vi "thermo_config_dialog.vi"(8 "error in":errorcluster, 11 "thermo in":T1={"type"=enum."COMET Tx5xx (ethernet)", "comment"="", "tag"="", "refresh"=5.0, "IP"="", "port"=502, "VISA"="", "last readout"=timestamp(0 s since 1904-01-01), "TCP ref"=refnum, "VISA sess"="", "idn"="", "press"=0.0, "RH"=0.0, "temp"=0.0, "pres cor"=[], "RH cor"=[], "temp cor"=[], "try left"=0, "failed"=FALSE, "RTD set"=[], "RTD inv"=[], "range"=0.0, "net mode"=enum."MODBUS", "try fail"=enum."Stop trying - return NaN", "timeout [s]"=0.0, "max retries"=0, "sim t [deg]"=0.0, "status"=0} {"status" items=["ok", "retry", "failed"]; "RTD inv" format="%.1f"; "RTD set" format="%.1f"; "temp cor" format="%.1f"; "RH cor" format="%.1f"; "pres cor" format="%.1f"; "refresh" min=0.1 max=1000.0 format="%.2f"}) -> (0 "error out":errorcluster, 3 "thermo out":T1={"type"=enum."COMET Tx5xx (ethernet)", "comment"="", "tag"="", "refresh"=5.0, "IP"="", "port"=502, "VISA"="", "last readout"=timestamp(0 s since 1904-01-01), "TCP ref"=refnum, "VISA sess"="", "idn"="", "press"=0.0, "RH"=0.0, "temp"=0.0, "pres cor"=[], "RH cor"=[], "temp cor"=[], "try left"=0, "failed"=FALSE, "RTD set"=[], "RTD inv"=[], "range"=0.0, "net mode"=enum."MODBUS", "try fail"=enum."Stop trying - return NaN", "timeout [s]"=0.0, "max retries"=0, "sim t [deg]"=0.0, "status"=0} {"status" items=["ok", "retry", "failed"]; "RTD inv" format="%.1f"; "RTD set" format="%.1f"; "temp cor" format="%.1f"; "RH cor" format="%.1f"; "pres cor" format="%.1f"; "refresh" min=0.1 max=1000.0 format="%.2f"})   [LabVIEW 2020]
doc: "Thermometer configuration dialogue."
uses:
  thermo_types.ctl
  Thermometer Config Tab Control.ctl
  Thermometer Fail Action.ctl
  RTD/RTD_preset.ctl
  thermo.ctl
  varilib/varilib.lvlib
panel:
  in  "btn default":bool caption="OK Button"
  in  "tc base":enum32{"Page"}(tab)
  in  "refresh":dbl=30.0 caption="Refresh rate [s]" min=0.0 max=1000.0 format="%#.2f"
  in  "comment":string="dummy thermometer" caption="Instrument comment"
  in  "tag":string="dut" caption="Instrument tag"
  in  "type":T2 caption="Type"
  in  "tc com":enum32{"Page"}(tab)
  in  "timeout":dbl=5.0 caption="Readout timeout [s]" min=0.1 max=30.0
  in  "retry N":i32=10 caption="Maximum readout tries" min=0 max=100
  in  "try fail":T3=enum."Stop trying - return NaN" caption="Retries failed action"
  in  "tc idn":enum32{"Page"}(tab)
  out "ID string":string
  out "temp":string caption="t [deg C]"
  out "RH":string caption="RH [%]"
  out "press":string caption="p [Pa]"
  out "RTD list":T4[](array[typedef]) {"tref" format="%.3f"; "Rref [Ohm]" format="%.3f"; "RTD poly" format="%_6e"}
  out "tc setup":T5
  in  "sim t [deg]":dbl caption="mean t [deg]"
  in  "temp cor":dbl[][](array[numeric]) caption="Temperature corrections [deg C]" format="%.1f"
  in  "IP":string="192.168.2.34" caption="IP address"
  in  "port":u16=502 caption="MODBUS port"
  in  "RH cor":dbl[][](array[numeric]) caption="RH corrections [%]" format="%.1f"
  in  "pres cor":dbl[][](array[numeric]) caption="Pressure corrections [Pa]" format="%.1f"
  in  "btn dmm auto":bool
  in  "tref [deg C]":dbl caption="t ref [deg C]" format="%.3f"
  in  "save btn":bool
  in  "R ref [Ohm]":dbl=100.0 format="%_6f"
  in  "VISA":refnum<visa-resource-name>
  in  "def btn":bool
  in  "rtd sens":u16(ring) caption="Default presets" items=["KT210", "KT210", "Pt100", "Pt1000", "Pt100_PT4"]
  in  "RTD poly":dbl[](array[numeric])=[1.0, 0.005485, 6.65e-06, 0.0, 2.805e-11, 0.0, -2e-17] caption="Polynome [deg C^-n]" format="%_6e"
  in  "load btn":bool
  in  "RTD name":string caption="New preset name"
  in  "range":dbl caption="Range [Ohm]" format="%#_6f"
  out "read ok":bool caption="READ"
  out "read fail":bool
  in  "btn cancel":bool
  in  "btn tst":bool
  in  "btn ok":bool
  # "ref. temp.:"
  # "correction:"
  # "ref. RH.:"
  # "correction:"
  # "ref. pres.:"
  # "correction:"
  # "RTD coefficients:"
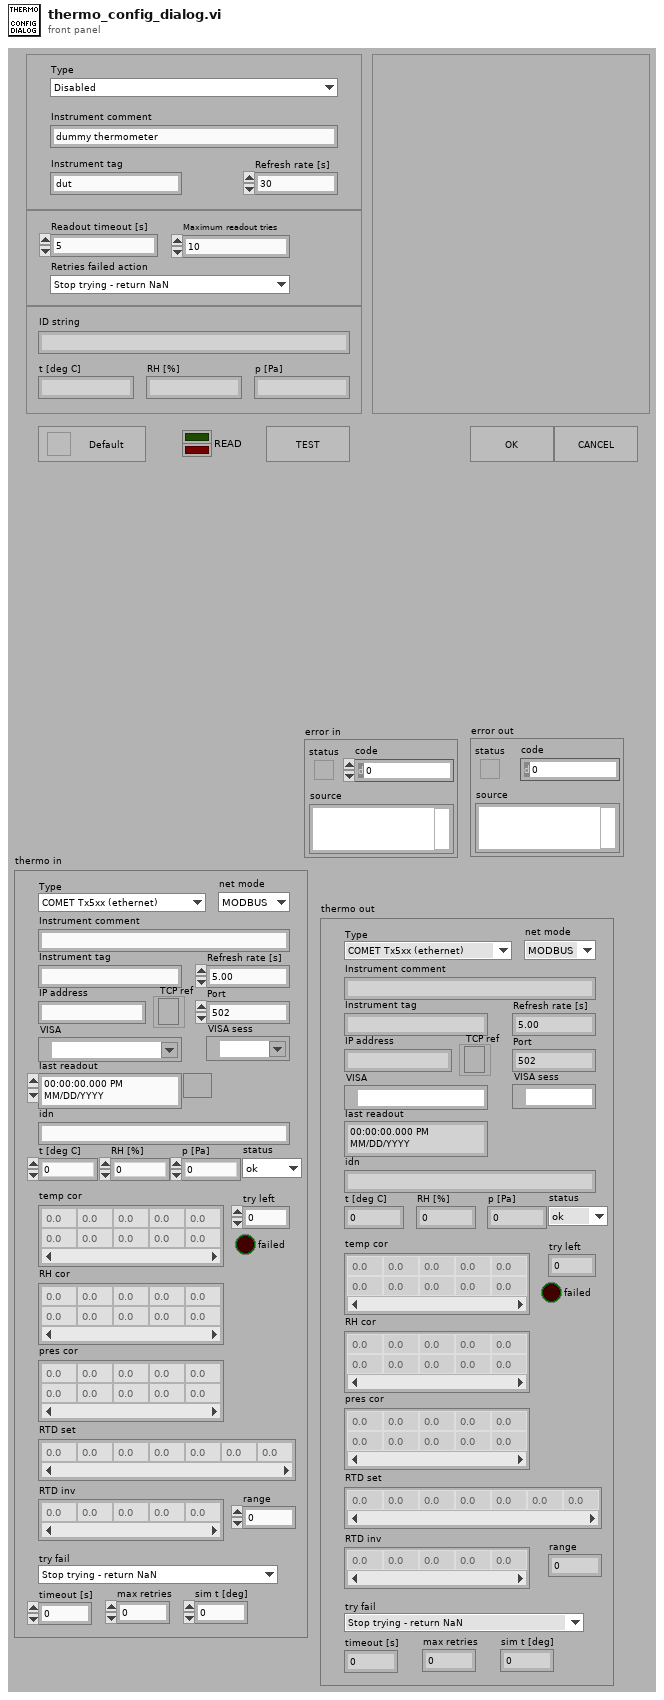
[diagram p1: front panel]
types:
  T1 = typedef "thermo.ctl" = cluster{"type":T2, "comment":string, "tag":string, "refresh":dbl, "IP":string, "port":u16, "VISA":refnum<visa-resource-name>, "last readout":timestamp, "TCP ref":refnum<k5>, "VISA sess":refnum<visa-resource-name>, "idn":string, "press":dbl, "RH":dbl, "temp":dbl, "pres cor":dbl[][], "RH cor":dbl[][], "temp cor":dbl[][], "try left":i32, "failed":bool, "RTD set":dbl[], "RTD inv":dbl[], "range":dbl, "net mode":enum16{"MODBUS", "HTTP"}, "try fail":T3, "timeout [s]":dbl, "max retries":i32, "sim t [deg]":dbl, "status":u16}
  T2 = typedef "thermo_types.ctl" = enum16{"Disabled", "Simulated", "COMET Tx5xx (ethernet)", "Keithley 2002 (GPIB) + RTD", "Agilent 344xx (GPIB) + RTD"}
  T3 = typedef "Thermometer Fail Action.ctl" = enum16{"Stop trying - keep last value", "Stop trying - return NaN", "Generate error - stop sweep"}
  T4 = typedef "RTD_preset.ctl" = cluster{"Rref [Ohm]":dbl, "tref":dbl, "RTD poly":dbl[], "name":string}
  T5 = typedef "Thermometer Config Tab Control.ctl" = enum32{"none", "sim", "COMET", "DMM"}
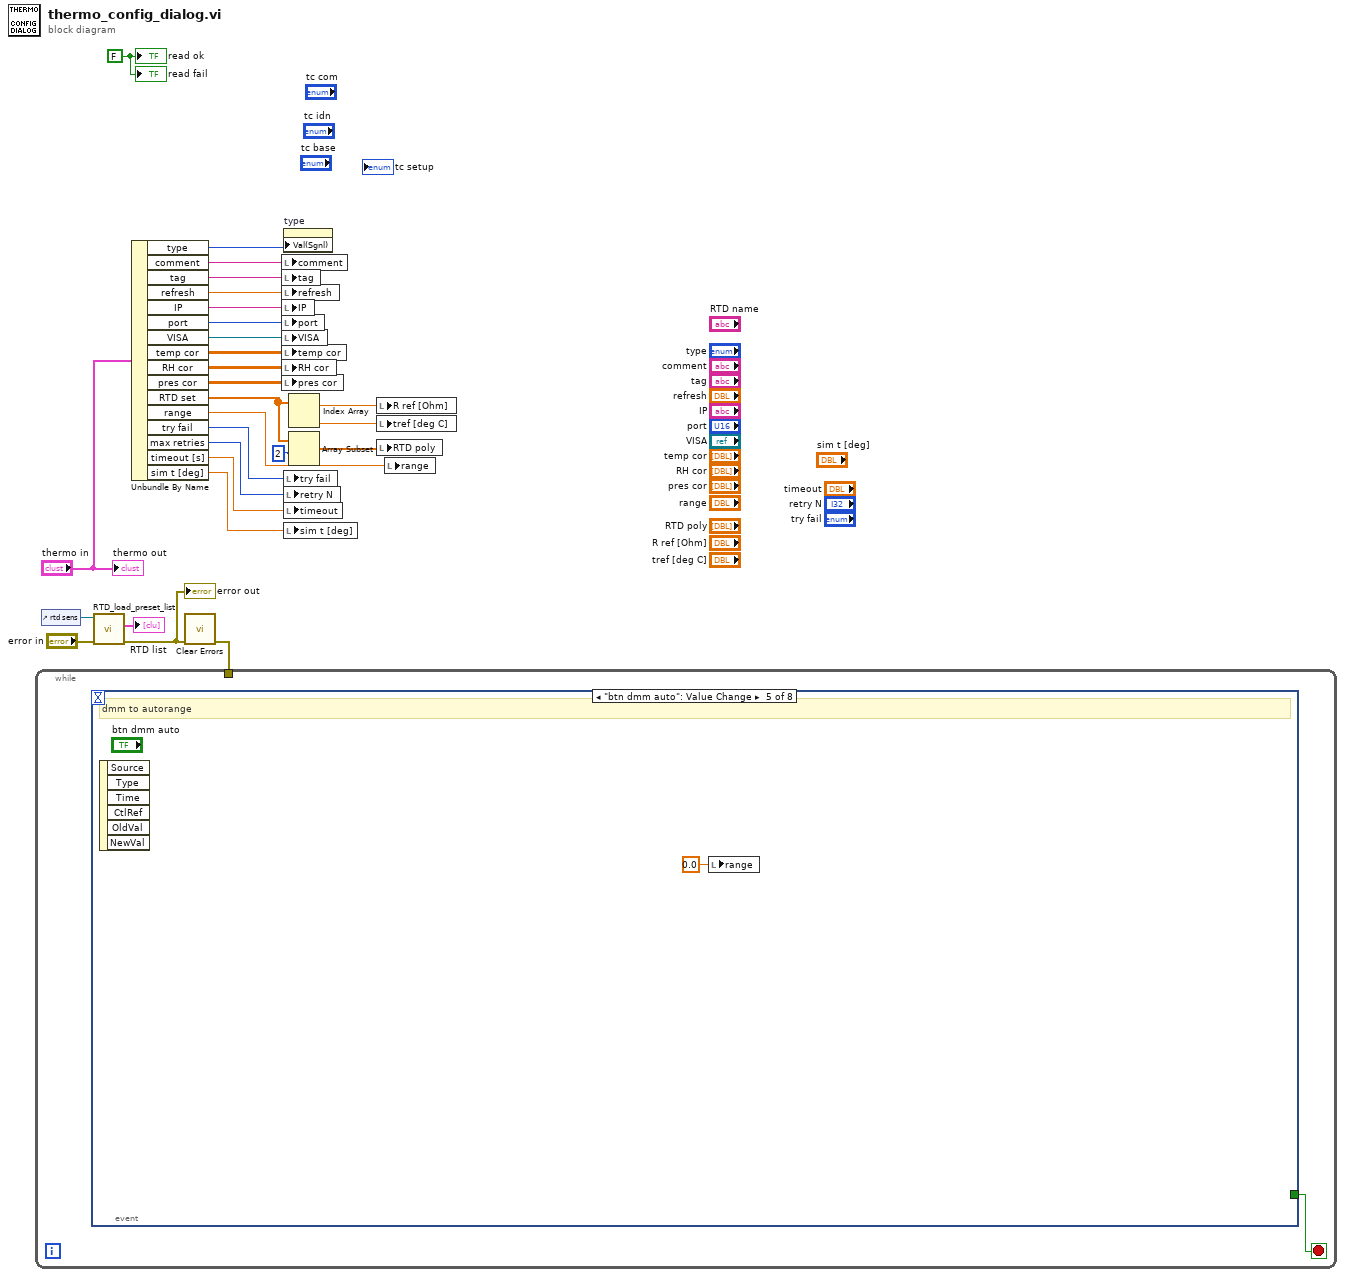
[diagram p0: block diagram]
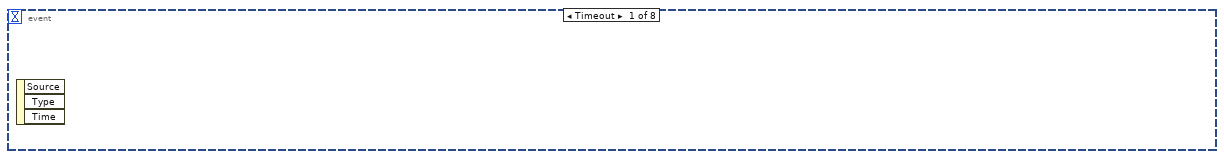
[diagram p2: hidden frame]
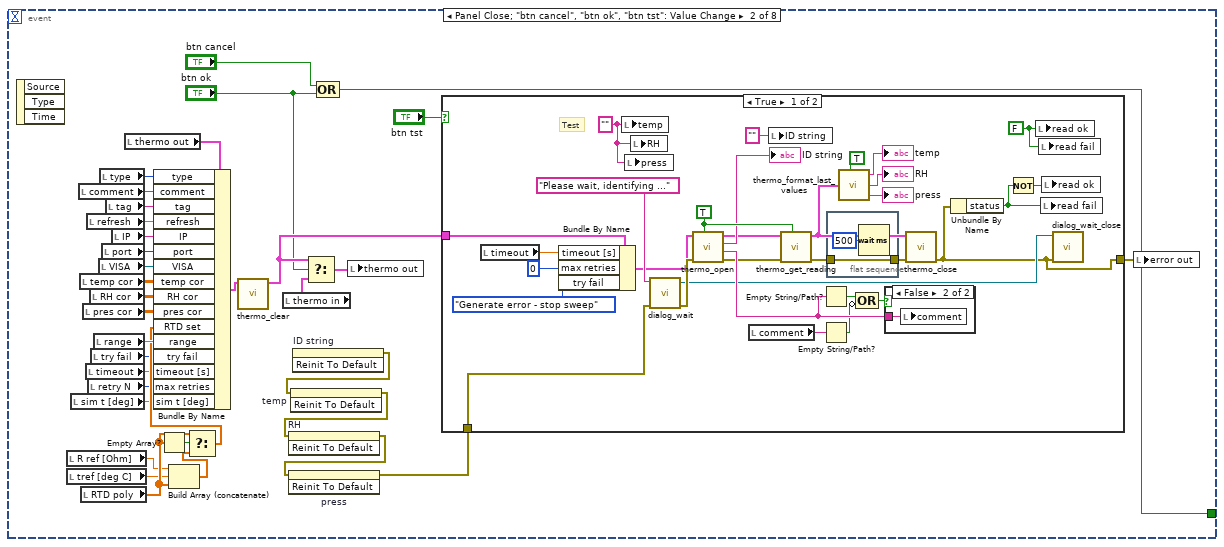
[diagram p3: hidden frame]
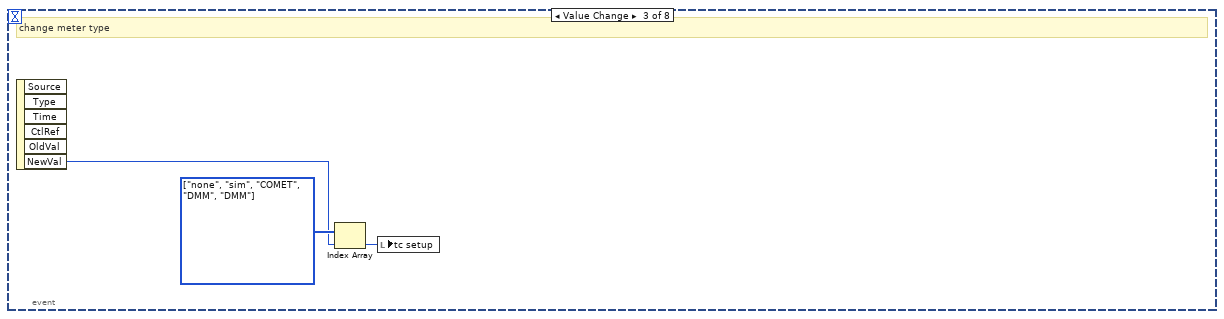
[diagram p6: hidden frame]
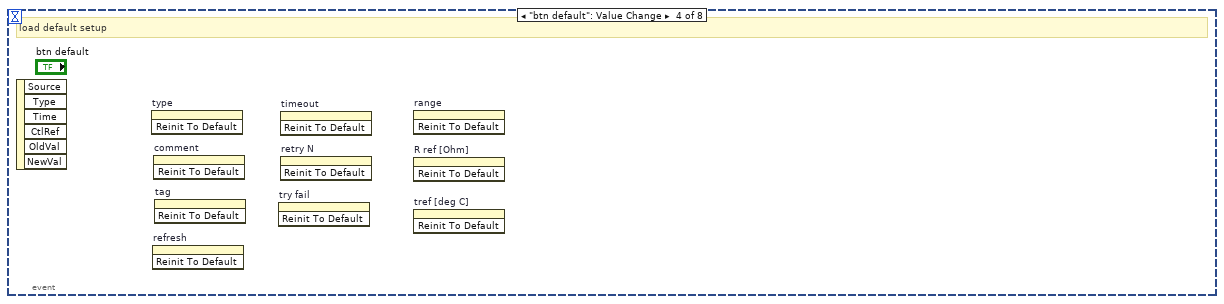
[diagram p7: hidden frame]
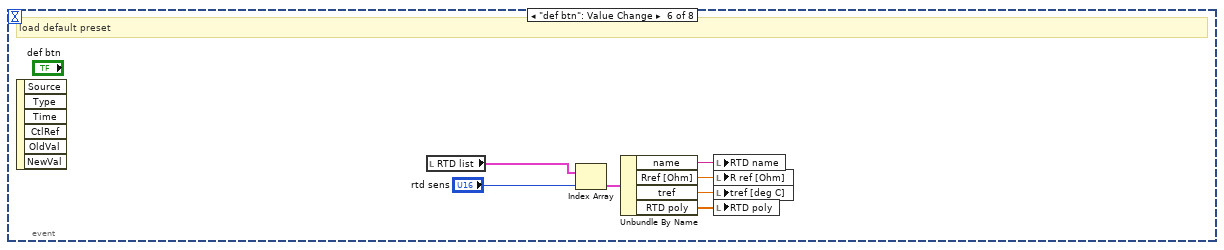
[diagram p8: hidden frame]
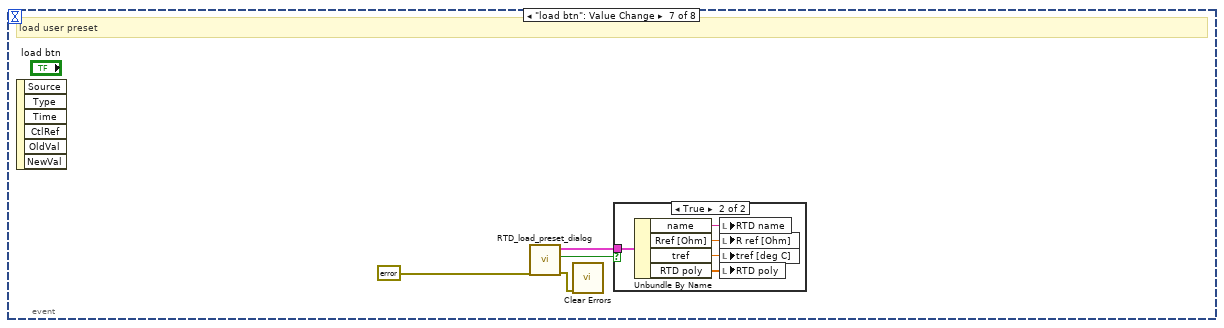
[diagram p9: hidden frame]
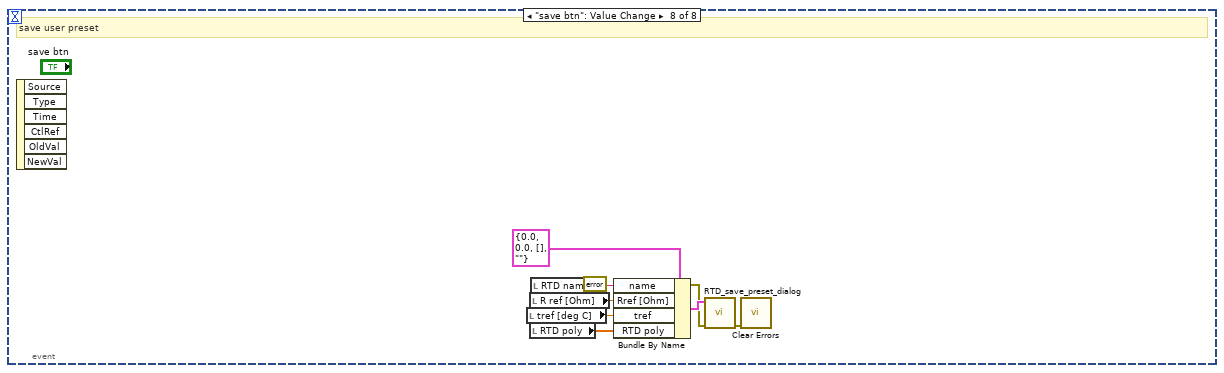
[diagram p11: hidden frame]
diagram:
  w27 = FALSE ("read ok")
  n1 = control-ref of="rtd sens"() -> (w26:refnum<vi>)
  n2 = call "RTD_load_preset_list.vi"("error in"="error in", "list ref in"=w26) -> ("error out"=w6:errorcluster, "list out"=→"RTD list":T4[])  [unwired: 6 in, 2 out]
  "error out" <- w6
  n3 = Unbundle By Name("thermo in") -> ("type"=w1:T2, "comment"=w22:string, "tag"=w21:string, "refresh"=w19:dbl, "IP"=w20:string, "port"=w18:u16, "VISA"=w17:refnum<visa-resource-name>, "temp cor"=w16:dbl[][], "RH cor"=w15:dbl[][], "pres cor"=w14:dbl[][], "RTD set"=w9:dbl[], "range"=w8:dbl, "try fail"=w4:T3, "max retries"=w3:i32, "timeout [s]"=w5:dbl, "sim t [deg]"=w2:dbl)
  n4 = call <vilib>:"Clear Errors.vi"("error in (no error)"=w6) -> ("error out"=w7:errorcluster)  [unwired: 5 in, 1 out]
  n5 = while {
    tunnel: w7 -> [_]
    stop <- w28 stop-if-true
    n6 = event shown="[4] \"btn dmm auto\": Value Change" {
      selector: _ -> [_ _ _ _ _ _ _ _]
      dyn-events: _ -> [_ _ _ _ _ _ _ _]
      timeout: _ -> [_ _ _ _ _ _ _ _]
      tunnel: [_ w29 _ _ _ _ _ _] -> w28
      event Timeout {
        n7 = event-data() -> ()  [unwired: 1 in, 3 out]
      }
      event Panel Close; "btn cancel", "btn ok", "btn tst": Value Change {
        n8 = event-data() -> ()  [unwired: 1 in, 3 out]
        n9 = local read "R ref [Ohm]"() -> (w60:dbl)
        n10 = local read "tref [deg C]"() -> (w62:dbl)
        n11 = local read "sim t [deg]"() -> (w32:dbl)
        n12 = local read "comment"() -> (w51:string)
        n13 = local read "temp cor"() -> (w58:dbl[][])
        n14 = local read "RTD poly"() -> (w63:dbl[])
        n15 = local read "pres cor"() -> (w59:dbl[][])
        n16 = local read "timeout"() -> (w40:dbl)
        n17 = local read "refresh"() -> (w53:dbl)
        n18 = local read "retry N"() -> (w39:i32)
        n19 = local read "RH cor"() -> (w57:dbl[][])
        n20 = local read "try fail"() -> (w41:T3)
        n21 = local read "range"() -> (w61:dbl)
        n22 = local read "VISA"() -> (w56:refnum<visa-resource-name>)
        n23 = local read "type"() -> (w50:T2)
        n24 = local read "port"() -> (w55:u16)
        n25 = local read "tag"() -> (w52:string)
        n26 = local read "IP"() -> (w54:string)
        n27 = local read "thermo out"() -> (w46:T1)
        n28 = Empty Array?(array=w63) -> (empty?=w47:bool)
        n29 = Build Array (concatenate)(w60, w62, w63) -> (w48:dbl[])
        n30 = Select(t=w63, s=w47, f=w48) -> (s? t:f=w49:dbl[])
        n31 = Bundle By Name(cluster=w46, "type"=w50, "comment"=w51, "tag"=w52, "refresh"=w53, "IP"=w54, "port"=w55, "VISA"=w56, "temp cor"=w58, "RH cor"=w57, "pres cor"=w59, "RTD set"=w49, "range"=w61, "try fail"=w41, "timeout [s]"=w40, "max retries"=w39, "sim t [deg]"=w32) -> (w38:T1)
        n32 = call "thermo_clear.vi"("thermo in"=w38) -> ("thermo out"=w37:T1)  [unwired: 9 in, 1 out]
        n33 = local read "thermo in"() -> (w44:T1)
        n34 = invoke on="ID string" class="Str" method="Reinit To Default"() -> (error out=w36:errorcluster)  [unwired: 3 in, 2 out]
        n35 = invoke on="temp" class="Str" method="Reinit To Default"(error in=w36) -> (error out=w35:errorcluster)  [unwired: 2 in, 2 out]
        n36 = invoke on="RH" class="Str" method="Reinit To Default"(error in=w35) -> (error out=w34:errorcluster)  [unwired: 2 in, 2 out]
        n37 = invoke on="press" class="Str" method="Reinit To Default"(error in=w34) -> (error out=w33:errorcluster)  [unwired: 2 in, 2 out]
        n38 = Select(t=w37, s="btn ok", f=w44) -> (s? t:f=w45:T1)
        n39 = Compound Arithmetic op=OR("btn cancel", "btn ok") -> (w29:bool)
        n40 = local write "thermo out"(w45) -> ()
        n41 = case shown="True" "btn tst" {
          tunnel: w37 -> [w71 _]
          tunnel: [w65 w98] -> w42
          tunnel: w33 -> [w66 w98]
          frame True {
            w84 = "" ("temp")
            w91 = FALSE ("read ok")
            w94 = TRUE ("force open")
            # "Test"
            n42 = local read "timeout"() -> (w68:dbl)
            n43 = Bundle By Name(cluster=w71, "timeout [s]"=w68, "max retries"=0 ("retry N in"), "try fail"=Thermometer_Fail_Action."Generate error - stop sweep") -> (w70:T1)
            n44 = local write "temp"(w84) -> ()
            n45 = local write "press"(w84) -> ()
            n46 = local write "RH"(w84) -> ()
            n47 = call "dialog_wait.vi"("error in"=w66, "message string"="Please wait, identifying ..." ("msg")) -> ("error out"=w78:errorcluster, "reference out"=w76:refnum<vi>)  [unwired: 8 in]
            n48 = call "thermo_open.vi"("force open"=w94, "error in"=w78, "thermo in"=w70) -> ("error out"=w64:errorcluster, "instrument name"=w88:string, "ID string"=→"ID string":string, "thermo out"=w72:T1)  [unwired: 5 in]
            n49 = local read "comment"() -> (w82:string)
            n50 = local write "ID string"("" ("ID string")) -> ()
            n51 = call "thermo_get_reading.vi"("force read"=w94, "error in"=w64, "thermo"=w72) -> ("error out"=w75:errorcluster, "thermo out"=w73:T1)  [unwired: 2 in, 5 out]
            n52 = Empty String/Path?(string/path=w88) -> (empty?=w80:bool)
            n53 = Empty String/Path?(string/path=w82) -> (empty?=w79:bool)
            n54 = flat-sequence {
              tunnel: w75 -> [w96]
              tunnel: [w96] -> w74
              frame #0 {
                n55 = Wait (ms)(milliseconds to wait=u32 500) -> ()  [unwired: 1 out]
              }
            }
            n56 = call "thermo_format_last_values.vi"("force print"=TRUE, "thermo"=w73) -> ("temperature"=→"temp":string, "RH"=→"RH":string, "pressure"=→"press":string)  [unwired: 3 in]
            n57 = Compound Arithmetic op=OR(w80, invert w79) -> (w81:bool)
            n58 = case shown="False" w81 {
              tunnel: w88 -> [_ w97]
              frame True {
              }
              frame False {
                n59 = local write "comment"(w97) -> ()
              }
            }
            n60 = call "thermo_close.vi"("error in"=w74, "thermo in"=w73) -> ("error out"=w65:errorcluster)  [unwired: 8 in, 1 out]
            n61 = Unbundle By Name(w65) -> ("status"=w93:bool)
            n62 = Not(x=w93) -> (.not. x?=w92:bool)
            n63 = local write "read ok"(w91) -> ()
            n64 = local write "read fail"(w91) -> ()
            n65 = local write "read fail"(w93) -> ()
            n66 = local write "read ok"(w92) -> ()
            n67 = call "dialog_wait_close.vi"("error in"=w65, "async vi ref"=w76) -> ()  [unwired: 2 in]
          }
          frame False {
          }
        }
        n68 = local write "error out"(w42) -> ()
      }
      event Value Change {
        w101 = T5[] [enum."none", enum."sim", enum."COMET", enum."DMM", enum."DMM"] items=["none", "sim", "COMET", "DMM"]
        # "change meter type"
        n69 = event-data() -> ("NewVal"=w99:T2)  [unwired: 1 in, 5 out]
        n70 = Index Array(array=w101, index=w99) -> (element=w100:T5)
        n71 = local write "tc setup"(w100) -> ()
      }
      event "btn default": Value Change {
        # "load default setup"
        n72 = event-data() -> ()  [unwired: 1 in, 6 out]
        n73 = invoke on="type" class="Enum (strict)" method="Reinit To Default"() -> ()  [unwired: 3 in, 3 out]
        n74 = invoke on="refresh" class="DigNum (strict)" method="Reinit To Default"() -> ()  [unwired: 3 in, 3 out]
        n75 = invoke on="comment" class="Str" method="Reinit To Default"() -> ()  [unwired: 3 in, 3 out]
        n76 = invoke on="tag" class="Str" method="Reinit To Default"() -> ()  [unwired: 3 in, 3 out]
        n77 = invoke on="try fail" class="Enum (strict)" method="Reinit To Default"() -> ()  [unwired: 3 in, 3 out]
        n78 = invoke on="timeout" class="DigNum (strict)" method="Reinit To Default"() -> ()  [unwired: 3 in, 3 out]
        n79 = invoke on="retry N" class="DigNum (strict)" method="Reinit To Default"() -> ()  [unwired: 3 in, 3 out]
        n80 = invoke on="range" class="DigNum (strict)" method="Reinit To Default"() -> ()  [unwired: 3 in, 3 out]
        n81 = invoke on="R ref [Ohm]" class="DigNum (strict)" method="Reinit To Default"() -> ()  [unwired: 3 in, 3 out]
        n82 = invoke on="tref [deg C]" class="DigNum (strict)" method="Reinit To Default"() -> ()  [unwired: 3 in, 3 out]
      }
      event "btn dmm auto": Value Change {
        # "dmm to autorange"
        n83 = event-data() -> ()  [unwired: 1 in, 6 out]
        n84 = local write "range"(0.0 ("range")) -> ()
      }
      event "def btn": Value Change {
        # "load default preset"
        n85 = event-data() -> ()  [unwired: 1 in, 6 out]
        n86 = local read "RTD list"() -> (w104:T4[])
        n87 = Index Array(array=w104, index="rtd sens") -> (element=w105:T4)
        n88 = Unbundle By Name(w105) -> ("name"=w108:string, "Rref [Ohm]"=w106:dbl, "tref"=w109:dbl, "RTD poly"=w107:dbl[])
        n89 = local write "RTD name"(w108) -> ()
        n90 = local write "R ref [Ohm]"(w106) -> ()
        n91 = local write "tref [deg C]"(w109) -> ()
        n92 = local write "RTD poly"(w107) -> ()
      }
      event "load btn": Value Change {
        # "load user preset"
        n93 = event-data() -> ()  [unwired: 1 in, 6 out]
        n94 = call "RTD_load_preset_dialog.vi"("error in"=errorcluster {"status"=FALSE, "code"=0, "source"=""}) -> ("error out"=w111:errorcluster, "successfull"=w113:bool, "preset"=w112:T4)  [unwired: 7 in, 1 out]
        n95 = call <vilib>:"Clear Errors.vi"("error in (no error)"=w111) -> ()  [unwired: 5 in, 2 out]
        n96 = case shown="True" w113 {
          tunnel: w112 -> [_ w114]
          frame False {
          }
          frame True {
            n97 = Unbundle By Name(w114) -> ("name"=w118:string, "Rref [Ohm]"=w116:dbl, "tref"=w115:dbl, "RTD poly"=w117:dbl[])
            n98 = local write "RTD name"(w118) -> ()
            n99 = local write "R ref [Ohm]"(w116) -> ()
            n100 = local write "tref [deg C]"(w115) -> ()
            n101 = local write "RTD poly"(w117) -> ()
          }
        }
      }
      event "save btn": Value Change {
        # "save user preset"
        n102 = event-data() -> ()  [unwired: 1 in, 6 out]
        n103 = local read "tref [deg C]"() -> (w119:dbl)
        n104 = local read "R ref [Ohm]"() -> (w125:dbl)
        n105 = local read "RTD poly"() -> (w124:dbl[])
        n106 = local read "RTD name"() -> (w126:string)
        n107 = Bundle By Name(cluster=T4 {"Rref [Ohm]"=0.0, "tref"=0.0, "RTD poly"=[], "name"=""} ("preset"), "name"=w126, "Rref [Ohm]"=w125, "tref"=w119, "RTD poly"=w124) -> (w122:T4)
        n108 = call "RTD_save_preset_dialog.vi"("error in"=errorcluster {"status"=FALSE, "code"=0, "source"=""}, "preset"=w122) -> ("error out"=w120:errorcluster)  [unwired: 9 in]
        n109 = call <vilib>:"Clear Errors.vi"("error in (no error)"=w120) -> ()  [unwired: 5 in, 2 out]
      }
    }
  }
  n110 = local write "comment"(w22) -> ()
  n111 = local write "tag"(w21) -> ()
  n112 = local write "refresh"(w19) -> ()
  n113 = local write "IP"(w20) -> ()
  n114 = local write "port"(w18) -> ()
  n115 = local write "VISA"(w17) -> ()
  n116 = local write "temp cor"(w16) -> ()
  n117 = local write "RH cor"(w15) -> ()
  n118 = local write "pres cor"(w14) -> ()
  n119 = property on="type" class="Enum (strict)"("Val(Sgnl)"=w1) -> ()  [unwired: 2 in, 2 out]
  n120 = local write "try fail"(w4) -> ()
  n121 = local write "retry N"(w3) -> ()
  n122 = local write "timeout"(w5) -> ()
  n123 = local write "sim t [deg]"(w2) -> ()
  n124 = Index Array(array=w9) -> (element #1=w12:dbl, element #2=w11:dbl)  [unwired: 2 in]
  n125 = Array Subset(array=w9, index=2) -> (w10:dbl[])  [unwired: 1 in]
  n126 = local write "R ref [Ohm]"(w12) -> ()
  n127 = local write "tref [deg C]"(w11) -> ()
  n128 = local write "RTD poly"(w10) -> ()
  n129 = local write "range"(w8) -> ()
  "read fail" <- w27
  "read ok" <- w27
  "thermo out" <- "thermo in"
